vi "UnloadAction.vi"(8 "error in (no error)":errorcluster caption="entrée d'erreur (pas d'erreur)", 11 "MultiHarp In":refnum<class "MultiHarp150.lvclass"> caption="DNL_LabVIEW Object in") -> (0 "error out":errorcluster caption="sortie d'erreur", 3 "MultiHarp Out":refnum<class "MultiHarp150.lvclass"> caption="DNL_LabVIEW Object out")   [LabVIEW 2019, in "MultiHarp150.lvclass"]
uses:
  MultiHarp150.lvclass
  C:/Programmes Labview/LabscanV1A/DevicesClass/BaseDevice/BaseDevice.lvclass
  MultiHarp150.lvclass/MultiHarp150.ctl
  BaseDevice/BaseDevice.lvclass
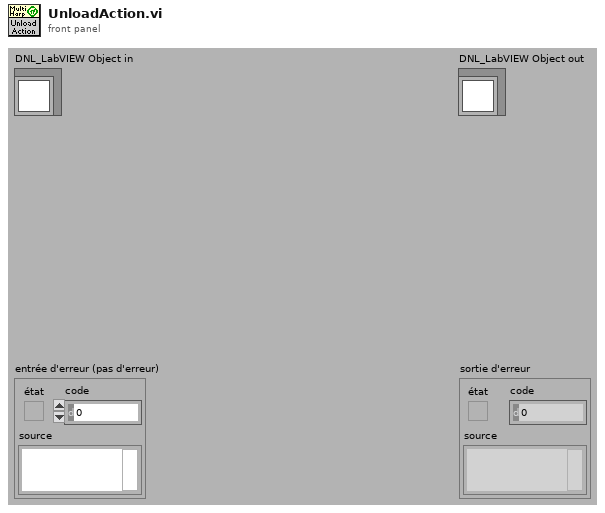
[diagram p1: front panel]
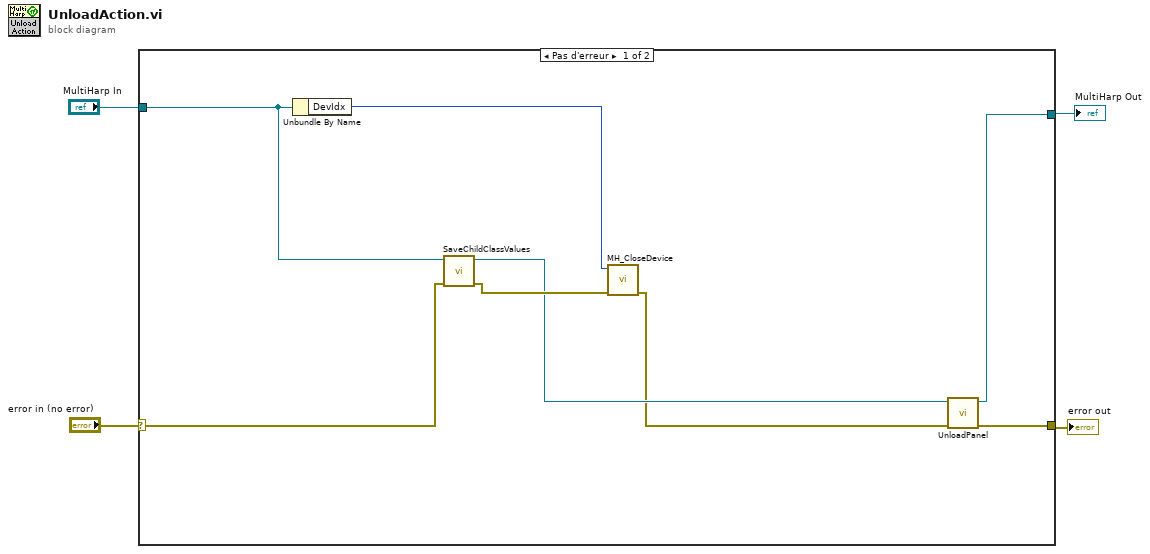
[diagram p0: block diagram]
diagram:
  n1 = case shown="Pas d'erreur" "error in (no error)" {
    selector: "error in (no error)" -> [w10 w13]
    tunnel: [w12 w13] -> w3
    tunnel: [w11 w14] -> w2
    tunnel: "MultiHarp In" -> [w9 w14]
    frame No Error {
      n2 = Unbundle By Name(w9) -> ("DevIdx"=w8:i32)
      n3 = call "SaveChildClassValues.vi"("error in (no error)"=w10, "MultiHarp150 en entrée"=w9) -> ("error out"=w7:errorcluster, "MultiHarp150 en sortie"=w6:refnum<class "MultiHarp150.lvclass">)  [unwired: 8 in]
      n4 = call <userlib>:"MH_CloseDevice.vi"("error in (no error)"=w7, "devidx"=w8) -> ("error out"=w5:errorcluster)  [unwired: 8 in, 1 out]
      n5 = call "UnloadPanel.vi"("error in (no error)"=w5, "Device en entrée"=w6) -> ("error out"=w12:errorcluster, "Device en sortie"=w11:refnum<class "MultiHarp150.lvclass">)  [unwired: 8 in]
    }
    frame Error {
    }
  }
  "error out" <- w3
  "MultiHarp Out" <- w2
